vi "Get Column Info.vi"(8 "error in (no error)":errorcluster, 9 "Column Name Array (All)":string[](array[string]), 10 "Table Name":string, 11 "ODBC in":refnum<class "ADODB.lvclass">) -> (0 "error out":errorcluster, 2 "Column Information Array":T1[](array[typedef]), 3 "ODBC out":refnum<class "ADODB.lvclass">)   [LabVIEW 2020, in "ADODB.lvlib" / "ADODB.lvclass"]
uses:
  ADODB.lvclass
  Database Interfaces/Column Information.ctl
  Database Interfaces/Database data type.ctl
  ADODB.lvclass/ADODB.ctl
  <vilib>/addons/database/NI_Database_API.lvlib
  Database Interfaces.lvlib
  ADODB.lvlib
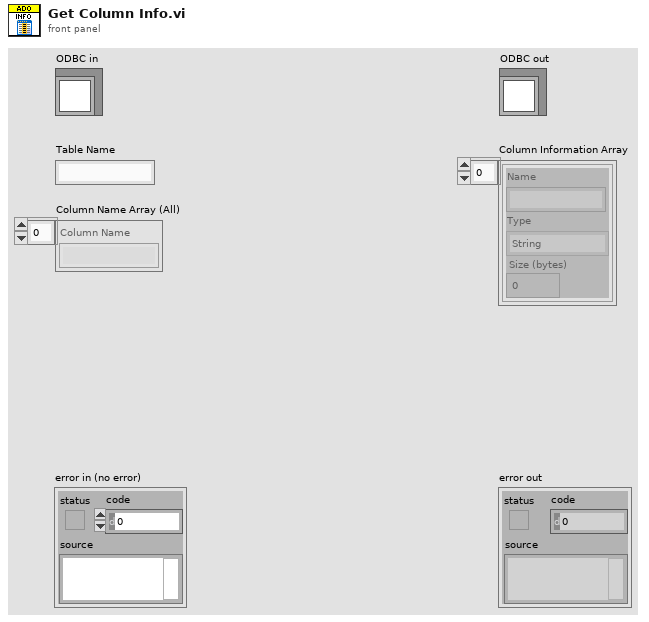
[diagram p1: front panel]
types:
  T1 = typedef "Database Interfaces.lvlib/Column Information.ctl" = cluster{"Name":string, "Type":T2, "Size (bytes)":i32}
  T2 = typedef "Database Interfaces.lvlib/Database data type.ctl" = enum16{"Undefined", "String", "Long (I32)", "Single (SGL)", "Double (DBL)", "Date/Time", "Binary"}
  T3 = typedef "NI_Database_API.lvlib/Conn ObjectReference.ctl" = refnum<k1>
  T4 = typedef "NI_Database_API.lvlib/DB Tools DataTypes.ctl" = enum16{"String", "Long (I32)", "Single (SGL)", "Double (DBL)", "Date/Time", "Binary"}
  T5 = cluster{"name":string, "database data type":T4, "defined size":i32}[]
  T6 = cluster{"name":string, "database data type":T4, "defined size":i32}
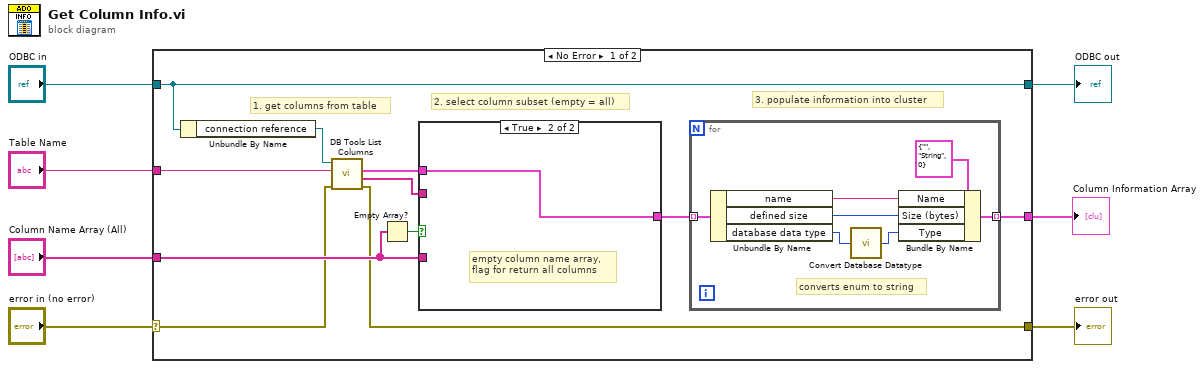
[diagram p0: block diagram]
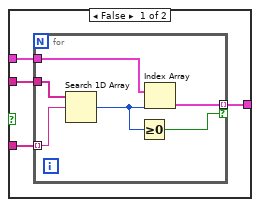
[diagram p2: hidden frame]
diagram:
  n1 = case shown="No Error" "error in (no error)" {
    selector: "error in (no error)" -> [w13 w38]
    tunnel: [w12 w38] -> w6
    tunnel: "ODBC in" -> [w17 w37]
    tunnel: [w17 w37] -> w4
    tunnel: "Table Name" -> [w16 _]
    tunnel: "Column Name Array (All)" -> [w14 _]
    tunnel: [w8 _] -> w1
    frame No Error {
      # "3. populate information into cluster"
      # "2. select column subset (empty = all)"
      # "1. get columns from table"
      n2 = Unbundle By Name(w17) -> ("connection reference"=w18:T3)
      n3 = call <vilib>:"DB Tools List Columns.vi"("error in (no error)"=w13, "table"=w16, "connection reference"=w18) -> ("error out"=w12:errorcluster, "columns"=w10:string[], "column information"=w11:T5)  [unwired: 1 in, 1 out]
      n4 = Empty Array?(array=w14) -> (empty?=w15:bool)
      n5 = case shown="True" w15 {
        tunnel: w14 -> [w29 _]
        tunnel: [w26 w36] -> w9
        tunnel: w11 -> [w27 w36]
        tunnel: w10 -> [w28 _]
        frame False {
          n6 = for {
            tunnel: w29 -> [w35] mode=indexing
            tunnel: w28 -> [w34]
            tunnel: w27 -> [w33]
            tunnel: [w32] -> w26 mode=indexing if=w30
            n7 = Search 1D Array(1D array=w34, element=w35) -> (index of element=w31:i32)  [unwired: 1 in]
            n8 = Greater Or Equal To 0?(x=w31) -> (x >= 0?=w30:bool)
            n9 = Index Array(array=w33, index=w31) -> (element=w32:T6)
          }
        }
        frame True {
          # "empty column name array,\nflag for return all columns"
        }
      }
      n10 = for {
        tunnel: w9 -> [w25] mode=indexing
        tunnel: [w22] -> w8 mode=indexing
        # "converts enum to string"
        n11 = Unbundle By Name(w25) -> ("name"=w24:string, "defined size"=w23:i32, "database data type"=w20:T4)
        n12 = call "Convert Database Datatype.vi"("ADODB data type"=w20) -> ("Database data type"=w19:T2)
        n13 = Bundle By Name(cluster=T1 {"Name"="", "Type"=enum."String", "Size (bytes)"=0} ("Column Information"), "Name"=w24, "Size (bytes)"=w23, "Type"=w19) -> (w22:T1)
      }
    }
    frame Error {
    }
  }
  "error out" <- w6
  "ODBC out" <- w4
  "Column Information Array" <- w1
